vi "Connection Close Tree.vi"(8 "error in (no error)":errorcluster, 11 "Connection DVR in":refnum<data-value>) -> (0 "error out":errorcluster, 3 "Connection DVR out":refnum<data-value>)   [LabVIEW 2015, in "MDSplus.lvlib"]
uses:
  <vilib>/MDSplus/Library/MDSplus.lvlib
  <vilib>/MDSplus/Classes/Connection_Class/Connection.lvclass
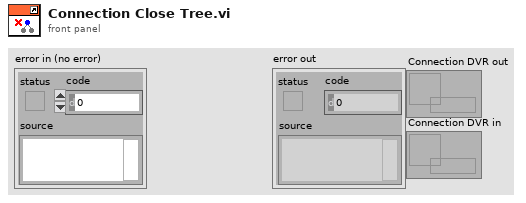
[diagram p1: front panel]
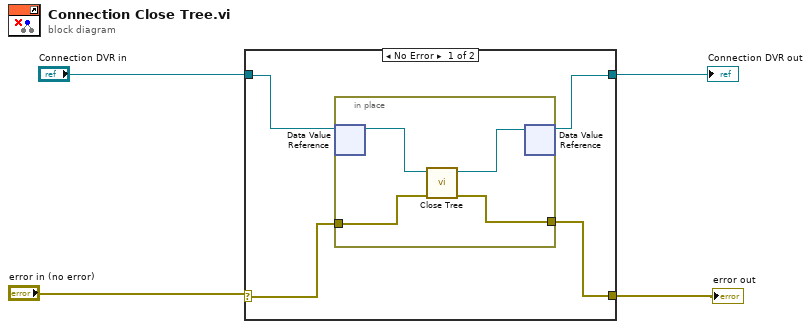
[diagram p0: block diagram]
diagram:
  n1 = case shown="No Error" "error in (no error)" {
    selector: "error in (no error)" -> [w6 w13]
    tunnel: "Connection DVR in" -> [w8 w14]
    tunnel: [w7 w14] -> w2
    tunnel: [w5 w13] -> w1
    frame No Error {
      n2 = in-place {
        in-place-border: w6 -> [w10]
        in-place-border: [w9] -> w5
        n3 = in-place-dvr #1(w8) -> (w12:refnum<class "Connection.lvclass">)  [unwired: 1 out]
        n4 = call <vilib>:"Close Tree.vi"("error in (no error)"=w10, "Connection in"=w12) -> ("error out"=w9:errorcluster, "Connection out"=w11:refnum<class "Connection.lvclass">)  [unwired: 8 in]
        n5 = in-place-dvr #1(w11) -> (w7:refnum<data-value>)  [unwired: 1 out]
      }
    }
    frame Error {
    }
  }
  "error out" <- w1
  "Connection DVR out" <- w2
